vi "TestShutter.vi"(0 "Open Time":sgl=1.0 min=0.1 format="%.2f") -> ()   [LabVIEW 2014]
panel:
  in  "Cycle Shutter":bool
  in  "Close Shutter":bool
  in  "Open Shutter":bool
  out "Open":bool
  in  "Exit":bool
  in  "Interval":sgl=3.0 min=1 format="%.2f"
  in  "Normally":bool=TRUE
  out "Cycle":i32
  # "secs"
  # "secs"
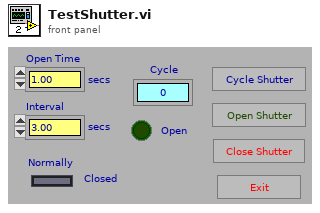
[diagram p1: front panel]
types:
  T1 = enum16{"OPEN", "CLOSE", "STATE_OPEN", "STATE_CLOSE"}
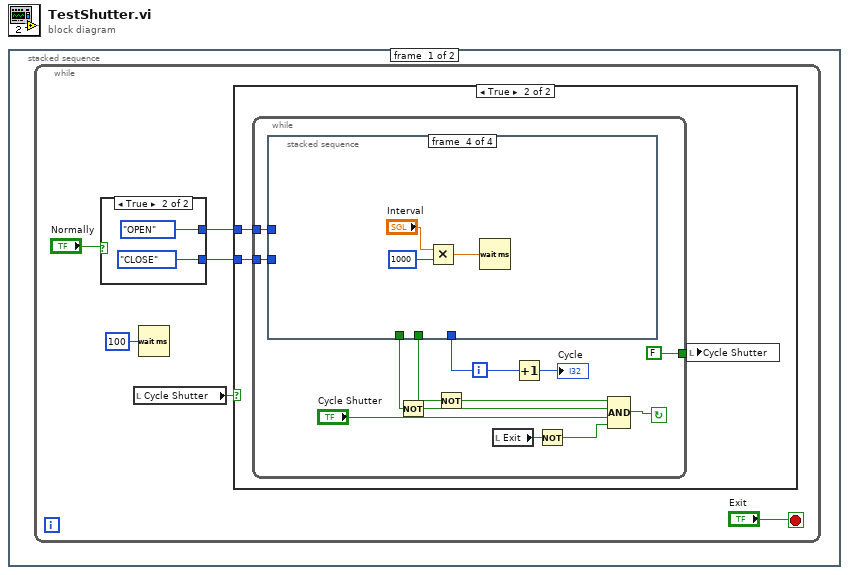
[diagram p0: block diagram]
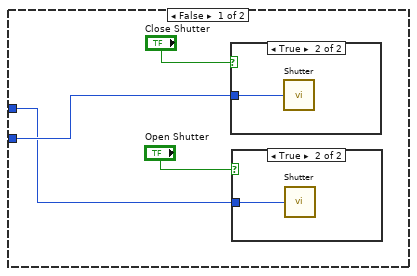
[diagram p2: hidden frame]
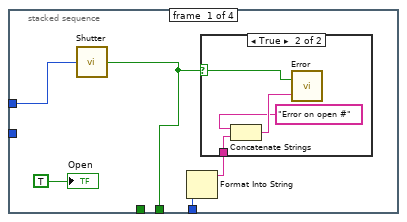
[diagram p5: hidden frame]
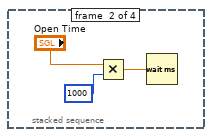
[diagram p7: hidden frame]
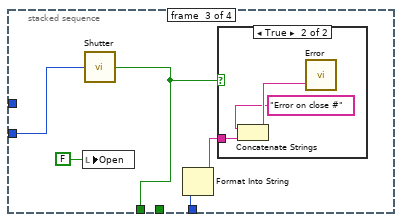
[diagram p8: hidden frame]
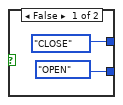
[diagram p10: hidden frame]
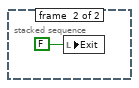
[diagram p11: hidden frame]
diagram:
  n1 = stacked-sequence {
    frame #0 {
      n2 = while {
        stop <- "Exit" stop-if-true
        n3 = case shown="True" "Normally" {
          tunnel: [T1."CLOSE" ("Shutter") T1."OPEN" ("Shutter")] -> w5
          tunnel: [T1."OPEN" ("Shutter") T1."CLOSE" ("Shutter")] -> w4
          frame False {
          }
          frame True {
          }
        }
        n4 = local read "Cycle Shutter"() -> (w3:bool)
        n5 = Wait (ms)(milliseconds to wait=u32 100) -> ()  [unwired: 1 out]
        n6 = case shown="True" w3 {
          tunnel: w5 -> [w7 w15]
          tunnel: w4 -> [w8 w14]
          frame False {
            n7 = case shown="True" "Close Shutter" {
              tunnel: w8 -> [_ w12]
              frame False {
              }
              frame True {
                n8 = call "Shutter.vi"("Shutter"=w12) -> ()  [unwired: 1 out]
              }
            }
            n9 = case shown="True" "Open Shutter" {
              tunnel: w7 -> [_ w11]
              frame False {
              }
              frame True {
                n10 = call "Shutter.vi"("Shutter"=w11) -> ()  [unwired: 1 out]
              }
            }
          }
          frame True {
            n11 = while {
              tunnel: w15 -> [w28]
              tunnel: w14 -> [w27]
              tunnel: [FALSE ("Stop")] -> w13
              i -> [w25]
              stop <- w22 continue-if-true
              n12 = stacked-sequence {
                tunnel: w25 -> [w33 _ w44 _]
                tunnel: w28 -> [w31 _ _ _]
                tunnel: w27 -> [_ _ w43 _]
                tunnel: [w29 _ _ _] -> w21
                tunnel: [_ _ w41 _] -> w20
                frame #0 {
                  n13 = call "Shutter.vi"("Shutter"=w31) -> ("Error"=w29:bool)
                  n14 = Format Into String(w33) -> (resulting string=w32:string)  [unwired: 3 in, 1 out]
                  n15 = case shown="True" w29 {
                    selector: w29 -> [_ w34]
                    tunnel: w32 -> [_ w37]
                    frame False {
                    }
                    frame True {
                      n16 = Concatenate Strings("Error on open #" ("Substring"), w37) -> (w36:string)
                      n17 = call "Error.vi"("Error String"=w36, "Error In"=w34) -> ()  [unwired: 1 in, 1 out]
                    }
                  }
                  "Open" <- TRUE ("Open")
                }
                frame #1 {
                  n18 = Multiply(x="Open Time", y=1000) -> (x*y=w39:sgl)
                  n19 = Wait (ms)(milliseconds to wait=w39) -> ()  [unwired: 1 out]
                }
                frame #2 {
                  n20 = local write "Open"(FALSE ("Open")) -> ()
                  n21 = call "Shutter.vi"("Shutter"=w43) -> ("Error"=w41:bool)
                  n22 = Format Into String(w44) -> (resulting string=w45:string)  [unwired: 3 in, 1 out]
                  n23 = case shown="True" w41 {
                    tunnel: w45 -> [_ w46]
                    frame False {
                    }
                    frame True {
                      n24 = Concatenate Strings("Error on close #" ("Substring"), w46) -> (w48:string)
                      n25 = call "Error.vi"("Error String"=w48) -> ()  [unwired: 2 in, 1 out]
                    }
                  }
                }
                frame #3 {
                  n26 = Multiply(x="Interval", y=u32 1000) -> (x*y=w49:sgl)
                  n27 = Wait (ms)(milliseconds to wait=w49) -> ()  [unwired: 1 out]
                }
              }
              n28 = Not(x=w20) -> (.not. x?=w17:bool)
              n29 = Not(x=w21) -> (.not. x?=w16:bool)
              n30 = local read "Exit"() -> (w19:bool)
              n31 = Increment(x=w25) -> (x+1=→"Cycle":i32)
              n32 = Not(x=w19) -> (.not. x?=w18:bool)
              n33 = Compound Arithmetic op=AND(w16, w17, "Cycle Shutter", w18) -> (w22:bool)
            }
            n34 = local write "Cycle Shutter"(w13) -> ()
          }
        }
      }
    }
    frame #1 {
      n35 = local write "Exit"(FALSE ("Exit")) -> ()
    }
  }
